vi "Include_when_Saving.vi"(8 "error in (no error)":errorcluster, 11 "AB_Source in":refnum<class "AB_Source.lvclass">) -> (0 "error out":errorcluster, 2 "include":bool, 3 "AB_Source out":refnum<class "AB_Source.lvclass">)   [LabVIEW 2020, in "AB_Source.lvclass"]
uses:
  <vilib>/AppBuilder/AB_Classes/Source/AB_Source.lvclass
  <vilib>/AppBuilder/AB_Classes/Source/AB_Source.lvclass/AB_Source.ctl
  <vilib>/AppBuilder/AB_Source_Inclusion.ctl
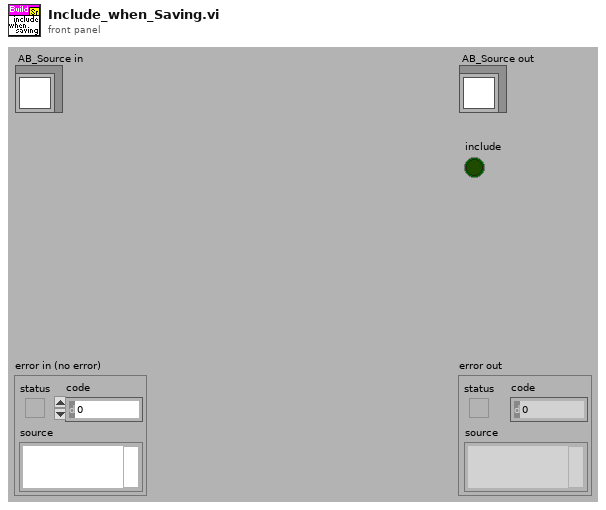
[diagram p1: front panel]
types:
  T1 = typedef "AB_Source_Inclusion.ctl" = enum16{"IncludeIfReferenced", "Include", "Exclude", "TopLevel"}
  T2 = typedef "AB_Source_Properties.ctl" = cluster{"sourcePropertyType":T3, "value":variant}
  T3 = typedef "AB_Source_Property_Type.ctl" = enum16{"Remove block diagram", "Remove front panel", "Password", "Window has title bar", "Show menu bar", "Show vertical scroll bar", "Show horizontal scroll bar", "Show toolbar", "Show Abort button", "Show fp when called", "Window behavior", "Allow user to close window", "Window run-time position", "Run when opened", "Allow debugging", "Auto error handling", "Generate guard code", "Use stack variables", "Expression folding", "Integer only", "Inline subVI"}
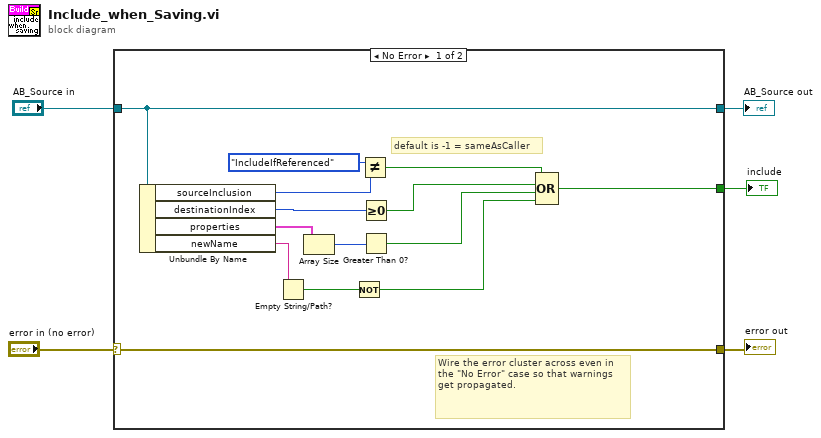
[diagram p0: block diagram]
diagram:
  n1 = case shown="No Error" "error in (no error)" {
    selector: "error in (no error)" -> [w19 w21]
    tunnel: [w19 w21] -> w4
    tunnel: [w18 w20] -> w2
    tunnel: "AB_Source in" -> [w18 w20]
    tunnel: [w11 _] -> w1
    frame No Error {
      # "default is -1 = sameAsCaller"
      # "Wire the error cluster across even in the \"No Error\" case so that warnings get propagated."
      n2 = Unbundle By Name(w18) -> ("sourceInclusion"=w17:T1, "destinationIndex"=w10:i32, "properties"=w14:T2[], "newName"=w8:string)
      n3 = Empty String/Path?(string/path=w8) -> (empty?=w7:bool)
      n4 = Array Size(array=w14) -> (size(s)=w13:i32)
      n5 = Not(x=w7) -> (.not. x?=w6:bool)
      n6 = Not Equal?(x=AB_Source_Inclusion."IncludeIfReferenced" ("y"), y=w17) -> (x != y?=w15:bool)
      n7 = Greater Or Equal To 0?(x=w10) -> (x >= 0?=w9:bool)
      n8 = Greater Than 0?(x=w13) -> (x > 0?=w12:bool)
      n9 = Compound Arithmetic op=OR(w15, w9, w12, w6) -> (w11:bool)
    }
    frame Error {
    }
  }
  "error out" <- w4
  "AB_Source out" <- w2
  "include" <- w1
